vi "SVA 4MV5 PF AHMI ECL VGD.vi"() -> ()   [LabVIEW 2020]
uses:
  Estados.ctl
  <vilib>/vision/driver/NI_Vision_Acquisition_Software.lvlib
  <vilib>/userDefined/High Color/IMAQdx.ctl
  <vilib>/vision/Image Controls.llb/IMAQ Image.ctl
panel:
  out "x >= y?":bool
  out "Redondez":dbl
  out "error out":errorcluster
  out "Procesos":enum32{"Captura", "Reporte"}(tab)
  in  "OK Button":bool
  out "Vista frontal":T1(plugin-control)
  out "Vista superior":T1(plugin-control)
  out "Color":u32(colorbox)
  out "Analisis frontal":T1(plugin-control)
  out "Analisis superior":T1(plugin-control)
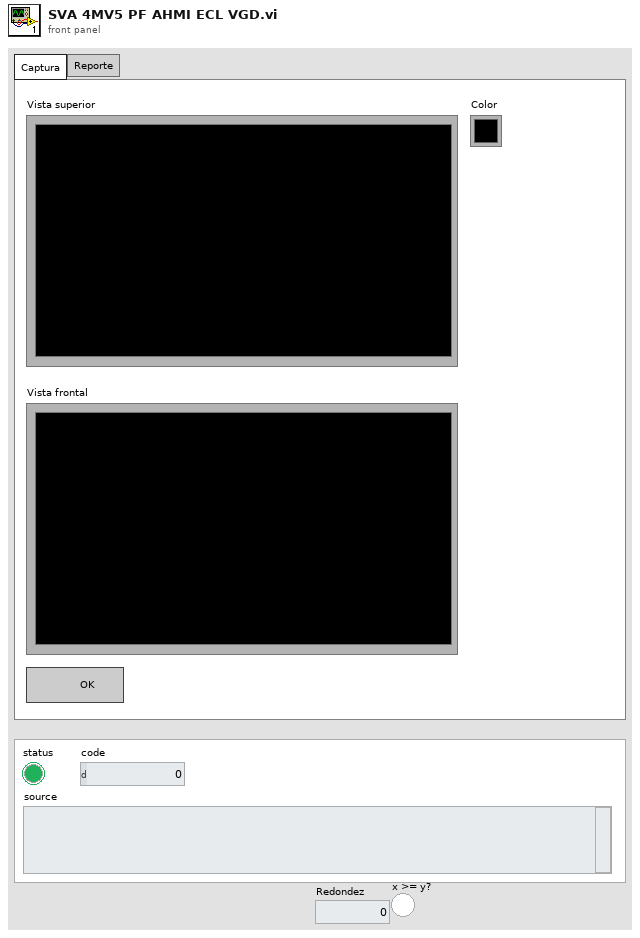
[diagram p1: front panel]
types:
  T1 = typedef "IMAQ Image.ctl" = refnum<image>
  T2 = typedef "Estados.ctl" = enum16{"Inicio", "Captura", "Procesamiento", "Reporte", "Fin"}
  T3 = typedef "IMAQdx.ctl" = refnum<k21>
  T4 = cluster{"Error":errorcluster, "Estados":T2, "frontal":T3, "superior":T3, "FRONTAL":T1, "SUPERIOR":T1, "Rfront":cluster{"Left":i32, "Top":i32, "Right":i32, "Bottom":i32}, "Rsup":cluster{"Left":i32, "Top":i32, "Right":i32, "Bottom":i32}}
  T5 = typedef "Image Type" = u32
  T6 = cluster{"Left":i32, "Top":i32, "Right":i32, "Bottom":i32}
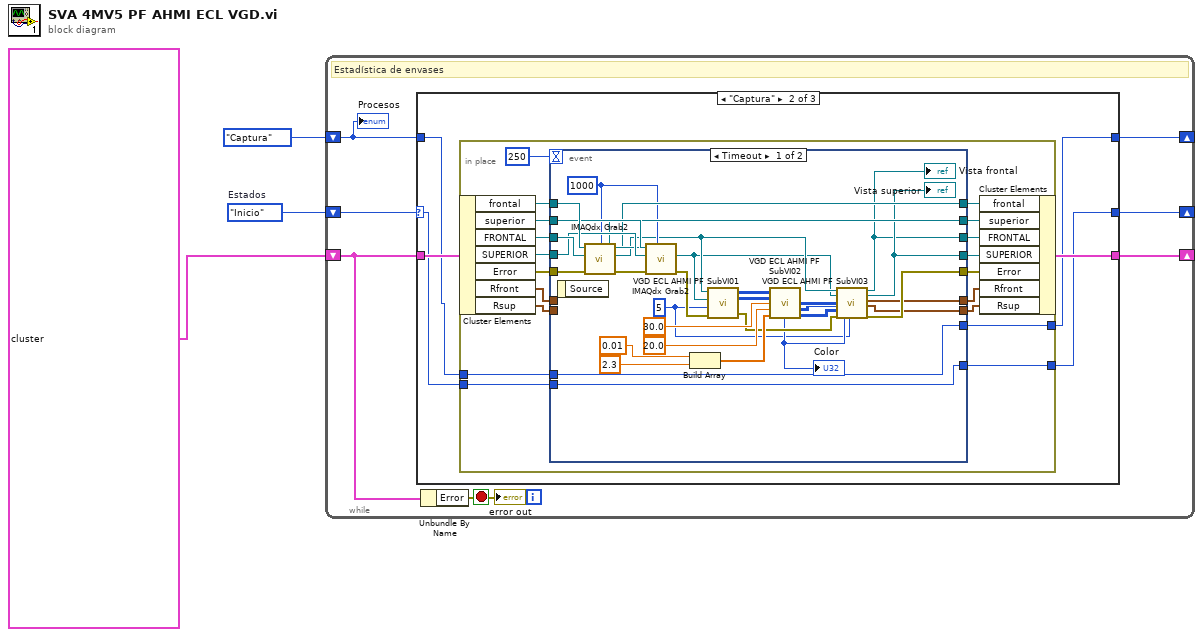
[diagram p0: block diagram]
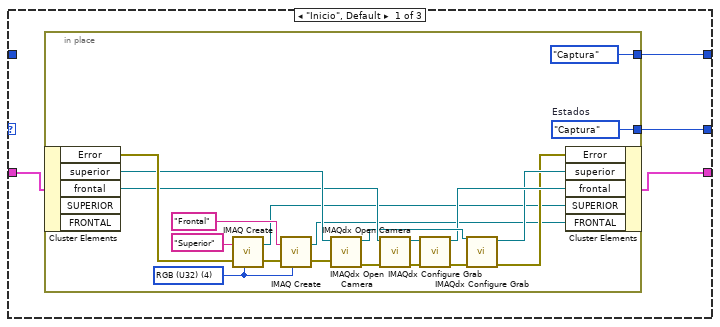
[diagram p2: hidden frame]
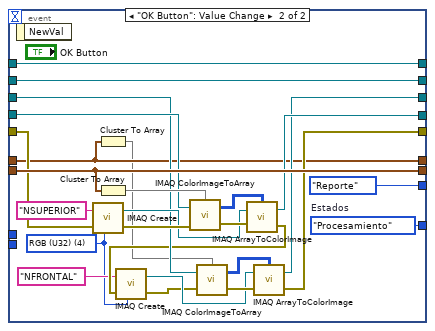
[diagram p3: hidden frame]
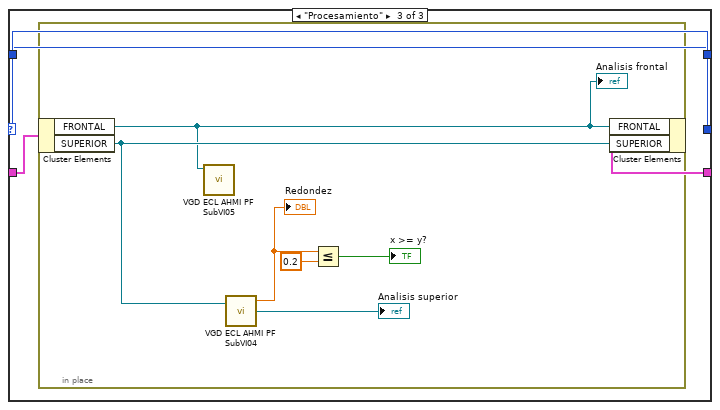
[diagram p4: hidden frame]
diagram:
  w2 = Estados."Inicio"  # Estados
  n1 = while {
    shift-right: [w7] -> _
    shift-left: T4 {"Error"={"status"=FALSE, "code"=0, "source"=""}, "Estados"=enum."Inicio", "frontal"="cam1", "superior"="cam2", "FRONTAL"=refnum, "SUPERIOR"=refnum, "Rfront"={"Left"=0, "Top"=0, "Right"=0, "Bottom"=0}, "Rsup"={"Left"=0, "Top"=0, "Right"=0, "Bottom"=0}} -> [w8]
    shift-right: [w6] -> _
    shift-left: w2 -> [w10]
    shift-right: [w5] -> _
    shift-left: enum32{"Captura", "Reporte"}."Captura" ("Procesos") -> [w4]
    stop <- w9 stop-if-true
    # "Estadística de envases"
    n2 = case shown="\"Captura\"" w10 {
      selector: w10 -> [_ w37 w120]
      tunnel: w8 -> [w14 w40 w119]
      tunnel: [w13 w39 w118] -> w7
      tunnel: [w12 w38 w120] -> w6
      tunnel: [w11 w36 w121] -> w5
      tunnel: w4 -> [_ w35 w121]
      frame "Inicio", Default {
        n3 = in-place {
          in-place-border: [w16] -> w12
          in-place-border: [enum32{"Captura", "Reporte"}."Captura" ("Procesos")] -> w11
          w16 = Estados."Captura"  # Estados
          w30 = T5 4 items=["Grayscale (U8)", "Grayscale (I16)", "Grayscale (SGL)", "Complex (CSG)", "RGB (U32)", "HSL (U32)", "RGB (U64)", "Grayscale (U16)"] ("Image Type")
          n4 = in-place-cluster #1(w14) -> ("Error"=w32:errorcluster, "superior"=w28:T3, "frontal"=w26:T3)  [unwired: 2 out]
          n5 = call "IMAQ Create"("Image Name"="Superior", "Image Type"=w30, "error in (no error)"=w32) -> ("New Image"=w18:T1, "error out"=w31:errorcluster)  [unwired: 2 in]
          n6 = call "IMAQ Create"("Image Name"="Frontal", "Image Type"=w30, "error in (no error)"=w31) -> ("New Image"=w17:T1, "error out"=w29:errorcluster)  [unwired: 2 in]
          n7 = call <vilib>:"IMAQdx Open Camera.vi"("error in"=w29, "Session In"=w28) -> ("error out"=w27:errorcluster, "Session Out"=w22:T3)  [unwired: 8 in]
          n8 = call <vilib>:"IMAQdx Open Camera.vi"("error in"=w27, "Session In"=w26) -> ("error out"=w25:errorcluster, "Session Out"=w23:T3)  [unwired: 8 in]
          n9 = call <vilib>:"IMAQdx Configure Grab.vi"("error in"=w25, "Session In"=w23) -> ("error out"=w24:errorcluster, "Session Out"=w21:T3)  [unwired: 8 in]
          n10 = call <vilib>:"IMAQdx Configure Grab.vi"("error in"=w24, "Session In"=w22) -> ("error out"=w19:errorcluster, "Session Out"=w20:T3)  [unwired: 8 in]
          n11 = in-place-cluster #1("Error"=w19, "superior"=w20, "frontal"=w21, "SUPERIOR"=w18, "FRONTAL"=w17) -> (w13:T4)
        }
      }
      frame "Captura" {
        n12 = in-place {
          in-place-border: [w44] -> w38
          in-place-border: w37 -> [w43]
          in-place-border: [w42] -> w36
          in-place-border: w35 -> [w41]
          n13 = in-place-cluster #2(w40) -> ("frontal"=w58:T3, "superior"=w57:T3, "FRONTAL"=w56:T1, "SUPERIOR"=w55:T1, "Error"=w59:errorcluster, "Rfront"=w46:T6, "Rsup"=w45:T6)
          n14 = event shown="[0] Timeout" {
            selector: _ -> [_ _]
            dyn-events: _ -> [_ _]
            timeout: 250 -> [_ _]
            tunnel: w59 -> [w91 w107]
            tunnel: w58 -> [w90 w117]
            tunnel: w57 -> [w88 w116]
            tunnel: w56 -> [w87 w100]
            tunnel: w55 -> [w86 w106]
            tunnel: [w85 w116] -> w54
            tunnel: [w84 w117] -> w53
            tunnel: [w73 w101] -> w52
            tunnel: [w66 w105] -> w51
            tunnel: [w65 w99] -> w50
            tunnel: [w64 w93] -> w48
            tunnel: [w63 w111] -> w47
            tunnel: w46 -> [_ w93]
            tunnel: w45 -> [_ w111]
            tunnel: [w62 w115] -> w44
            tunnel: w43 -> [w62 _]
            tunnel: [w61 enum32{"Captura", "Reporte"}."Reporte" ("Procesos")] -> w42
            tunnel: w41 -> [w61 _]
            event Timeout {
              w67 = 5 ("Factor diezmado")
              w83 = 1000 ("Timeout (ms)")
              n15 = event-data() -> ()  [unwired: 1 in, 1 out]
              n16 = call <vilib>:"IMAQdx Grab2.vi"("Timeout (ms)"=w83, "error in"=w91, "Image In"=w87, "Session In"=w90) -> ("error out"=w89:errorcluster, "Image Out"=w69:T1, "Session Out"=w84:T3)  [unwired: 4 in, 1 out]
              n17 = call <vilib>:"IMAQdx Grab2.vi"("Timeout (ms)"=w83, "error in"=w89, "Image In"=w86, "Session In"=w88) -> ("error out"=w82:errorcluster, "Image Out"=w68:T1, "Session Out"=w85:T3)  [unwired: 4 in, 1 out]
              n18 = Build Array(0.01 ("alfa"), 2.3 ("alfa 2")) -> (w76:dbl[])
              n19 = call "VGD ECL AHMI PF SubVI01.vi"("error in"=w82, "Factor diezmado"=w67, "SUPERIOR"=w68, "FRONTAL"=w69) -> ("error out"=w74:errorcluster, "pixmap S"=w80:u32[][], "pixmap F"=w81:u32[][])
              n20 = call "VGD ECL AHMI PF SubVI02.vi"("pixmap F"=w81, "pixmap S"=w80, "S"=30.0, "V"=20.0, "alfa"=w76) -> ("pixmap COLOR"=w71:u32[][], "pixmap GF"=w60:u32[][], "Color"=w72:u32, "pixmap GS"=w70:u32[][])  [unwired: 5 in, 2 out]
              "Color" <- w72
              n21 = call "VGD ECL AHMI PF SubVI03.vi"("FRONTAL"=w69, "SUPERIOR"=w68, "pixmap COLOR"=w71, "pixmap GF"=w60, "pixmap GS"=w70, "error in"=w74, "Color"=w72, "Factor diezmado"=w67) -> ("FRONTAL"=w65:T1, "SUPERIOR"=w66:T1, "Rfront"=w64:T6, "Rsup"=w63:T6, "error out"=w73:errorcluster)  [unwired: 7 in]
              "Vista frontal" <- w65
              "Vista superior" <- w66
            }
            event "OK Button": Value Change {
              w94 = T5 4 items=["Grayscale (U8)", "Grayscale (I16)", "Grayscale (SGL)", "Complex (CSG)", "RGB (U32)", "HSL (U32)", "RGB (U64)", "Grayscale (U16)"] ("Image Type")
              w115 = Estados."Procesamiento"  # Estados
              n22 = event-data() -> ()  [unwired: 1 in, 1 out]
              n23 = call "IMAQ Create"("Image Name"="NSUPERIOR", "Image Type"=w94, "error in (no error)"=w107) -> ("New Image"=w102:T1, "error out"=w113:errorcluster)  [unwired: 2 in]
              n24 = Cluster To Array(cluster=w93) -> (array=w92:i32[])
              n25 = Cluster To Array(cluster=w111) -> (array=w110:i32[])
              n26 = call "IMAQ ColorImageToArray"("Optional Rectangle"=w110, "Image"=w106, "error in (no error)"=w113) -> ("Image Pixels (U32)"=w108:u32[][], "error out"=w109:errorcluster)  [unwired: 1 in, 1 out]
              n27 = call "IMAQ ArrayToColorImage"("Image Pixels (U32)"=w108, "Image"=w102, "error in (no error)"=w109) -> ("Image Out"=w105:T1, "error out"=w96:errorcluster)  [unwired: 2 in]
              n28 = call "IMAQ Create"("Image Name"="NFRONTAL", "Image Type"=w94, "error in (no error)"=w96) -> ("New Image"=w98:T1, "error out"=w97:errorcluster)  [unwired: 2 in]
              n29 = call "IMAQ ColorImageToArray"("Optional Rectangle"=w92, "Image"=w100, "error in (no error)"=w97) -> ("Image Pixels (U32)"=w103:u32[][], "error out"=w104:errorcluster)  [unwired: 1 in, 1 out]
              n30 = call "IMAQ ArrayToColorImage"("Image Pixels (U32)"=w103, "Image"=w98, "error in (no error)"=w104) -> ("Image Out"=w99:T1, "error out"=w101:errorcluster)  [unwired: 2 in]
            }
          }
          n31 = in-place-cluster #2("frontal"=w53, "superior"=w54, "FRONTAL"=w50, "SUPERIOR"=w51, "Error"=w52, "Rfront"=w48, "Rsup"=w47) -> (w39:T4)
        }
      }
      frame "Procesamiento" {
        n32 = in-place {
          n33 = in-place-cluster #3(w119) -> ("FRONTAL"=w122:T1, "SUPERIOR"=w126:T1)
          "Analisis frontal" <- w122
          n34 = call "VGD ECL AHMI PF SubVI05.vi"("FRONTAL"=w122) -> ()  [unwired: 11 in]
          n35 = call "VGD ECL AHMI PF SubVI04.vi"("SUPERIOR"=w126) -> ("Redondez"=w125:dbl, "Analisis superior"=→"Analisis superior":T1)  [unwired: 1 in, 1 out]
          "Redondez" <- w125
          n36 = Less Or Equal?(x=w125, y=0.2) -> (x <= y?=→"x >= y?":bool)
          n37 = in-place-cluster #3("FRONTAL"=w122, "SUPERIOR"=w126) -> (w118:T4)
        }
      }
    }
    n38 = Unbundle By Name(w8) -> ("Error"=w9:errorcluster)
    "error out" <- w9
    "Procesos" <- w4
  }
